vi "TryUpdateAccelerometerSample.vi"   [LabVIEW 2016]
uses:
  <vilib>/Platform/TimedLoop/XDataNode/timing_clust.ctl
  <vilib>/Platform/TimedLoop/XDataNode/nitl_modes.ctl
  <vilib>/Platform/TimedLoop/XDataNode/wakeup.ctl
  Telemetry/TelemetryDataTypes.ctl
  Telemetry/TelemetryUpdateModes.ctl
  Telemetry/TelemetryFields.ctl
  <vilib>/rvi/Emulation/niFpgaEmulationIsFPGAContextNoSignature.vi
  <vilib>/rvi/Emulation/niFpgaSctlEmulationGetInTimedLoop.vi
  <vilib>/rvi/errors/niFpgaSetErrorForExecOnDevCompSimple.vi
  <vilib>/rvi/eio/common/nirviEmuReportErrorAndStop.vi
  <vilib>/rvi/DataTransferAndStorage/Container/Common/niFpgaContainerGetUniqueNameForEmu.vi
  <vilib>/rvi/FIFO/Fifo_Resource/nirvififoEmulationSetSize.vi
  <vilib>/rvi/FIFO/Fifo_Resource/nirviFifoEmulationQueueMgr.vi
  <instcachedir>/0/nirviFifoEmulationQueueMgr_E5CAEC123FF24DC58D834DCA3CDAA9B5.lvgen/nirviFifoEmulationQueueMgr_E5CAEC123FF24DC58D834DCA3CDAA9B5_026.vi
  <vilib>/Utility/error.llb/Clear Errors.vi
  <vilib>/rvi/FIFO/Fifo_Resource/nirvififoEmulationCreateLock.vi
  <vilib>/rvi/Emulation/niFpgaProcessEmulError.vi
  <vilib>/rvi/FIFO/Fifo_Resource/nirvififoEmulationObtainLock.vi
  <vilib>/rvi/FIFO/Fifo_Resource/nirvififoEmulationReleaseLock.vi
  <vilib>/rvi/occurrence/nirviWaitOnOccurrenceBase.vi
  <vilib>/rvi/errors/nirviReportUnexpectedCaseInternalError.vi
  <vilib>/rvi/errors/nirviReportUnexpectedCaseInternalError (U32).vi
  <vilib>/rvi/Emulation/niFpgaEmulationReportErrorSimple.vi
  <vilib>/rvi/Emulation/niFpgaGetClockAttributes.vi
  <vilib>/rvi/Emulation/niFpgaCriticalErrorInLSC.vi
  <instcachedir>/0/nirviFifoEmulationQueueMgr_E5CAEC123FF24DC58D834DCA3CDAA9B5.lvgen/nirviFifoEmulationQueueMgr_E5CAEC123FF24DC58D834DCA3CDAA9B5_038.vi
  <vilib>/rvi/FIFO/Fifo_Resource/nirvififoEmulationDetermineInputValidOut.vi
  <instcachedir>/0/nirviFifoEmulationQueueMgr_E5CAEC123FF24DC58D834DCA3CDAA9B5.lvgen/nirviFifoEmulationQueueMgr_E5CAEC123FF24DC58D834DCA3CDAA9B5_039.vi
  <vilib>/rvi/Memory/Memory_Emulation/niFpgaMemoryEmulationCacheClearOnFirstRun.vi
  <vilib>/rvi/Memory/Memory_Emulation/nirvimemoryEmulationManagerCache_MakeExclusive.vi
  <vilib>/rvi/Memory/Memory_Emulation/niFpgaMemoryEmulationValidateCache.vi
  <vilib>/rvi/Memory/Memory_Emulation/nirvimemoryEmulationManagerCache_InsertValue.vi
  <vilib>/rvi/Memory/Memory_Emulation/nirvimemoryEmulationManagerCache_ReleaseExclusive.vi
  <vilib>/rvi/Memory/Memory_Emulation/nirvimemoryEmulationManagerCache_GetValue.vi
  <vilib>/rvi/Memory/Memory_Emulation/nirvimemoryEmulationManagerCache_SetValue.vi
  <instcachedir>/0/nirviFifoEmulationQueueMgr_E5CAEC123FF24DC58D834DCA3CDAA9B5.lvgen/nirviFifoEmulationQueueMgr_E5CAEC123FF24DC58D834DCA3CDAA9B5_004.vi
  <vilib>/rvi/DataTransferAndStorage/Container/XNode/niFpgaContainer.xnode
  <vilib>/rvi/FIFO/Fifo_Resource/nirvififoEmulationRead.vi
  <vilib>/Platform/TimedLoop/XDataNode/XDataNode.xnode
  <vilib>/rvi/FIFO/Fifo_Resource/nirvififoEmulationWrite.vi
  <vilib>/rvi/DataTransferAndStorage/Register/Emulation/niFpgaRegisterEmulation.vi
  <vilib>/Platform/TimedLoop/XDataNode/XDNodeRunTimeDep.lvlib
types:
  T1 = cluster{"Timestamp":u64, "Accelerometer1Voltage":sgl, "Accelerometer2Voltage":sgl, "Accelerometer3Voltage":sgl, "Accelerometer4Voltage":sgl, "Accelerometer5Voltage":sgl, "Accelerometer6Voltage":sgl, "Accelerometer7Voltage":sgl, "Accelerometer8Voltage":sgl, "Accelerometer1Acceleration":sgl, "Accelerometer2Acceleration":sgl, "Accelerometer3Acceleration":sgl, "Accelerometer4Acceleration":sgl, "Accelerometer5Acceleration":sgl, "Accelerometer6Acceleration":sgl, "Accelerometer7Acceleration":sgl, "Accelerometer8Acceleration":sgl, "AngularAccelerationX":sgl, "AngularAccelerationY":sgl, "AngularAccelerationZ":sgl}
  T2 = typedef "TelemetryFields.ctl" = enum16{"None", "InclinometerTxBytes", "InclinometerRxBytes", "InclinometerTxFrames", "InclinometerRxFrames", "InclinometerErrorTimestamp", "InclinometerErrorCode", "InclinometerSampleTimestamp", "InclinometerRawAngle", "InclinometerZenithAngle", "DisplacementTxBytes", "DisplacementRxBytes", "DisplacementTxFrames", "DisplacementRxFrames", "DisplacementErrorTimestamp", "DisplacementErrorCode", "DisplacementSampleTimestamp", "DisplacementRaw1", "DisplacementRaw2", "DisplacementRaw3", "DisplacementRaw4", "DisplacementRaw5", "DisplacementRaw6", "DisplacementRaw7", "DisplacementRaw8", "DisplacementEng1", "DisplacementEng2", "DisplacementEng3", "DisplacementEng4", "DisplacementEng5", "DisplacementEng6", "DisplacementEng7", "DisplacementEng8", "DisplacementPositionX", "DisplacementPositionY", "DisplacementPositionZ", "DisplacementRotationX", "DisplacementRotationY", "DisplacementRotationZ", "AccelerometerSampleCount", "AccelerometerSampleTimestamp", "AccelerometerRaw1", "AccelerometerRaw2", "AccelerometerRaw3", "AccelerometerRaw4", "AccelerometerRaw5", "AccelerometerRaw6", "AccelerometerRaw7", "AccelerometerRaw8", "AccelerometerEng1", "AccelerometerEng2", "AccelerometerEng3", "AccelerometerEng4", "AccelerometerEng5", "AccelerometerEng6", "AccelerometerEng7", "AccelerometerEng8", "AngularAccelerationX", "AngularAccelerationY", "AngularAccelerationZ", "GyroTxBytes", "GyroRxBytes", "GyroTxFrames", "GyroRxFrames", "GyroErrorTimestamp", "GyroErrorCode", "GyroSampleTimestamp", "AngularVelocityX", "AngularVelocityY", "AngularVelocityZ", "GyroStatus", "GyroSequenceNumber", "GyroTemperature", "GyroBITTimestamp", "GyroBIT0", "GyroBIT1", "GyroBIT2", "GyroBIT3", "GyroBIT4", "GyroBIT5", "GyroBIT6", "GyroBIT7"}
  T3 = typedef "TelemetryUpdateModes.ctl" = enum8{"=", "+", "-", "|"}
  T4 = typedef "TelemetryDataTypes.ctl" = enum8{"U8", "U16", "U32", "U64", "I8", "I16", "I32", "I64", "SGL"}
  T5 = typedef "XDNodeRunTimeDep.lvlib/timing_clust.ctl" = cluster{"Expected End [f-1]":u64, "Actual End [f-1]":u64, "Finished Late? [f-1]":bool, "Expected End [i-1]":u64, "Actual End [i-1]":u64, "Finished Late? [i-1]":bool, "Expected Start [i]":u64, "Actual Start [i]":u64, "Expected Start [f]":u64, "Actual Start [f]":u64, "Source Name":string, "Structure Name":string, "Period":i64, "Deadline":i64, "Offset":i64, "Start":i64, "Priority":i32, "Timeout":i32, "Mode":T6, "Wakeup Reason":T7, "Error":errorcluster, "Source Type":string, "Secondary Source Type":string, "Global End Time":u64, "Global Start Time":u64, "Frame Duration":u64, "Iteration Duration":u64, "Assigned CPU":i32, "I/O Scan Engine Mode":u32}
  T6 = typedef "XDNodeRunTimeDep.lvlib/nitl_modes.ctl" = enum32{"No Change", "Process missed periods, maintain original phase", "Discard missed periods, maintain original phase", "Process missed periods, ignore original phase", "Discard missed periods, ignore original phase"}
  T7 = typedef "XDNodeRunTimeDep.lvlib/wakeup.ctl" = enum32{"Normal", "Aborted", "Asynchronous wakeup", "Timing source error", "Timed loop error", "Timeout"}
  T8 = typedef "TelemetryUpdateData.ctl" = cluster{"DataType":T4, "Mode":T3, "Field":T2, "Data":u64}
  T9 = typedef "TelemetryUpdateDataSGL.ctl" = cluster{"Mode":T3, "Field":T2, "Data":sgl}
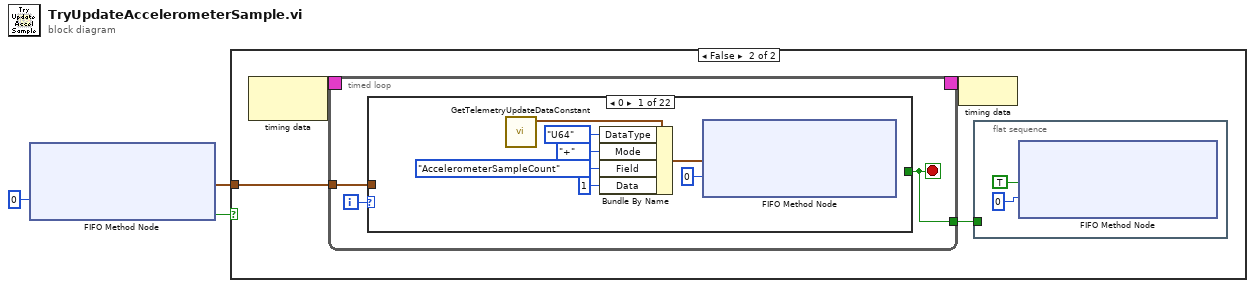
[diagram p0: block diagram]
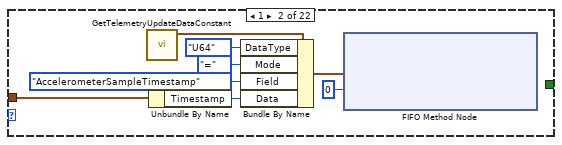
[diagram p3: hidden frame]
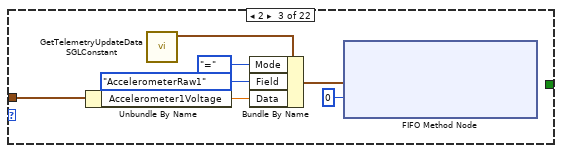
[diagram p4: hidden frame]
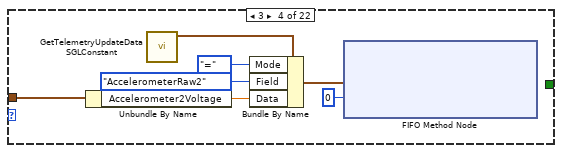
[diagram p5: hidden frame]
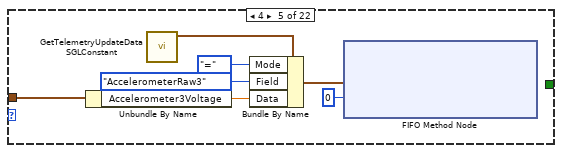
[diagram p6: hidden frame]
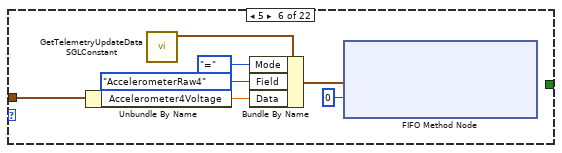
[diagram p7: hidden frame]
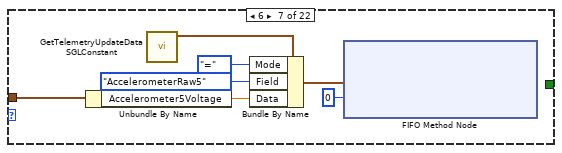
[diagram p8: hidden frame]
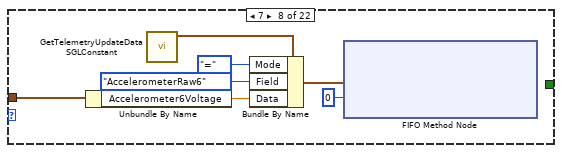
[diagram p9: hidden frame]
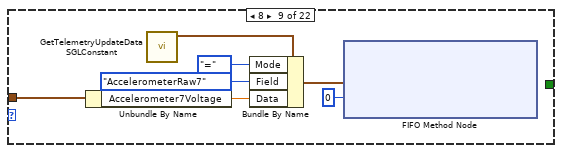
[diagram p10: hidden frame]
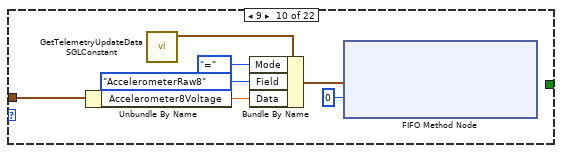
[diagram p11: hidden frame]
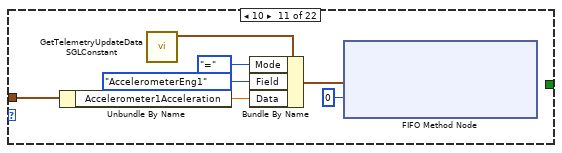
[diagram p12: hidden frame]
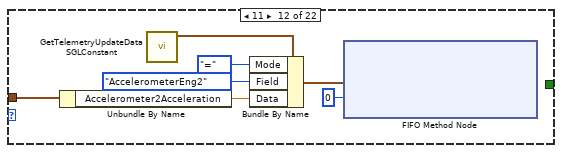
[diagram p13: hidden frame]
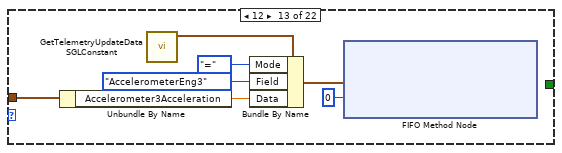
[diagram p14: hidden frame]
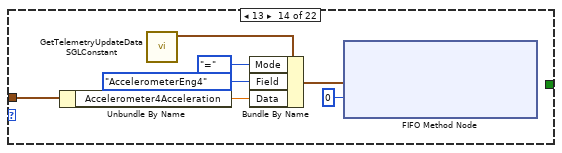
[diagram p15: hidden frame]
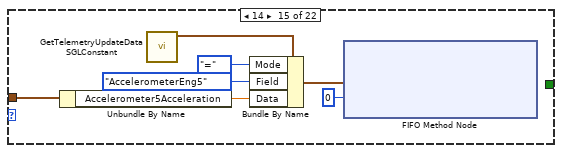
[diagram p16: hidden frame]
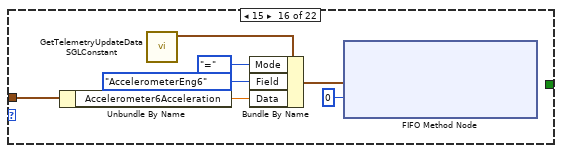
[diagram p17: hidden frame]
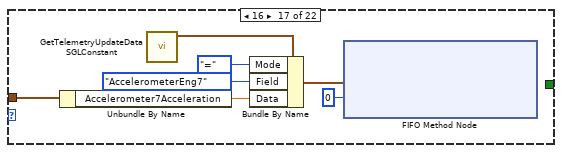
[diagram p18: hidden frame]
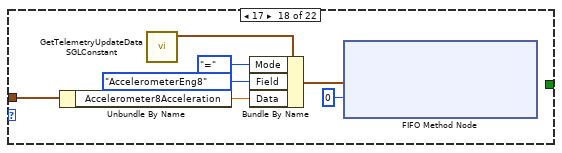
[diagram p19: hidden frame]
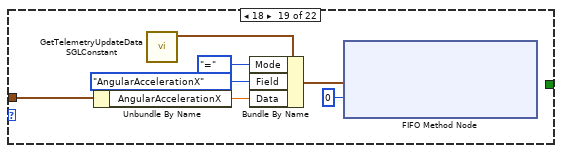
[diagram p20: hidden frame]
diagram:
  n1 = xnode ("FIFO Method Node")("Timeout"=0) -> ("Element"=w2:T1, "Timed Out?"=w3:bool)  [unwired: 1 in, 1 out]
  n2 = case shown="False" w3 {
    tunnel: w2 -> [_ w7]
    frame True {
    }
    frame False {
      n3 = node-c288() -> (w5:T5)  [unwired: 1 in]
      n4 = timed-loop {
        tunnel: w7 -> [w10]
        tunnel: [w9] -> w6
        timing: w5 -> [_]
        timing-out: [_] -> w4
        i -> [w8]
        stop <- w9 stop-if-true
        # "Move Data to Memory"
        n5 = case shown="0" w8 {
          tunnel: w10 -> [_ w19 w27 w34 w41 w48 w55 w62 w69 w76 w83 w90 w97 w104 w111 w118 w125 w132 w139 w146 w153 _]
          tunnel: [_ _ _ _ _ _ _ _ _ _ _ _ _ _ _ _ _ _ _ _ _ w159] -> w9
          frame 0 {
            n6 = call "GetTelemetryUpdateDataConstant.vi"() -> ("TelemetryUpdateData"=w16:T8)  [unwired: 11 in]
            n7 = Bundle By Name(cluster=w16, "DataType"=TelemetryDataTypes."U64" ("TelemetryDataTypes"), "Mode"=TelemetryUpdateModes."+" ("TelemetryUpdateModes"), "Field"=TelemetryFields."AccelerometerSampleCount" ("TelemetryFields"), "Data"=u64 1) -> (w14:T8)
            n8 = xnode ("FIFO Method Node")("Element"=w14, "Timeout"=0) -> ()  [unwired: 1 in, 2 out]
          }
          frame 1 {
            n9 = call "GetTelemetryUpdateDataConstant.vi"() -> ("TelemetryUpdateData"=w25:T8)  [unwired: 11 in]
            n10 = Unbundle By Name(w19) -> ("Timestamp"=w18:u64)
            n11 = Bundle By Name(cluster=w25, "DataType"=TelemetryDataTypes."U64" ("TelemetryDataTypes"), "Mode"=TelemetryUpdateModes."=" ("TelemetryUpdateModes"), "Field"=TelemetryFields."AccelerometerSampleTimestamp" ("TelemetryFields"), "Data"=w18) -> (w23:T8)
            n12 = xnode ("FIFO Method Node")("Element"=w23, "Timeout"=0) -> ()  [unwired: 1 in, 2 out]
          }
          frame 2 {
            n13 = Unbundle By Name(w27) -> ("Accelerometer1Voltage"=w26:sgl)
            n14 = call "GetTelemetryUpdateDataSGLConstant.vi"() -> ("TelemetryUpdateDataSGL"=w32:T9)  [unwired: 11 in]
            n15 = Bundle By Name(cluster=w32, "Mode"=TelemetryUpdateModes."=" ("TelemetryUpdateModes"), "Field"=TelemetryFields."AccelerometerRaw1" ("TelemetryFields"), "Data"=w26) -> (w30:T9)
            n16 = xnode ("FIFO Method Node")("Element"=w30, "Timeout"=0) -> ()  [unwired: 1 in, 2 out]
          }
          frame 3 {
            n17 = Unbundle By Name(w34) -> ("Accelerometer2Voltage"=w33:sgl)
            n18 = call "GetTelemetryUpdateDataSGLConstant.vi"() -> ("TelemetryUpdateDataSGL"=w39:T9)  [unwired: 11 in]
            n19 = Bundle By Name(cluster=w39, "Mode"=TelemetryUpdateModes."=" ("TelemetryUpdateModes"), "Field"=TelemetryFields."AccelerometerRaw2" ("TelemetryFields"), "Data"=w33) -> (w37:T9)
            n20 = xnode ("FIFO Method Node")("Element"=w37, "Timeout"=0) -> ()  [unwired: 1 in, 2 out]
          }
          frame 4 {
            n21 = Unbundle By Name(w41) -> ("Accelerometer3Voltage"=w40:sgl)
            n22 = call "GetTelemetryUpdateDataSGLConstant.vi"() -> ("TelemetryUpdateDataSGL"=w46:T9)  [unwired: 11 in]
            n23 = Bundle By Name(cluster=w46, "Mode"=TelemetryUpdateModes."=" ("TelemetryUpdateModes"), "Field"=TelemetryFields."AccelerometerRaw3" ("TelemetryFields"), "Data"=w40) -> (w44:T9)
            n24 = xnode ("FIFO Method Node")("Element"=w44, "Timeout"=0) -> ()  [unwired: 1 in, 2 out]
          }
          frame 5 {
            n25 = Unbundle By Name(w48) -> ("Accelerometer4Voltage"=w47:sgl)
            n26 = call "GetTelemetryUpdateDataSGLConstant.vi"() -> ("TelemetryUpdateDataSGL"=w53:T9)  [unwired: 11 in]
            n27 = Bundle By Name(cluster=w53, "Mode"=TelemetryUpdateModes."=" ("TelemetryUpdateModes"), "Field"=TelemetryFields."AccelerometerRaw4" ("TelemetryFields"), "Data"=w47) -> (w51:T9)
            n28 = xnode ("FIFO Method Node")("Element"=w51, "Timeout"=0) -> ()  [unwired: 1 in, 2 out]
          }
          frame 6 {
            n29 = Unbundle By Name(w55) -> ("Accelerometer5Voltage"=w54:sgl)
            n30 = call "GetTelemetryUpdateDataSGLConstant.vi"() -> ("TelemetryUpdateDataSGL"=w60:T9)  [unwired: 11 in]
            n31 = Bundle By Name(cluster=w60, "Mode"=TelemetryUpdateModes."=" ("TelemetryUpdateModes"), "Field"=TelemetryFields."AccelerometerRaw5" ("TelemetryFields"), "Data"=w54) -> (w58:T9)
            n32 = xnode ("FIFO Method Node")("Element"=w58, "Timeout"=0) -> ()  [unwired: 1 in, 2 out]
          }
          frame 7 {
            n33 = Unbundle By Name(w62) -> ("Accelerometer6Voltage"=w61:sgl)
            n34 = call "GetTelemetryUpdateDataSGLConstant.vi"() -> ("TelemetryUpdateDataSGL"=w67:T9)  [unwired: 11 in]
            n35 = Bundle By Name(cluster=w67, "Mode"=TelemetryUpdateModes."=" ("TelemetryUpdateModes"), "Field"=TelemetryFields."AccelerometerRaw6" ("TelemetryFields"), "Data"=w61) -> (w65:T9)
            n36 = xnode ("FIFO Method Node")("Element"=w65, "Timeout"=0) -> ()  [unwired: 1 in, 2 out]
          }
          frame 8 {
            n37 = Unbundle By Name(w69) -> ("Accelerometer7Voltage"=w68:sgl)
            n38 = call "GetTelemetryUpdateDataSGLConstant.vi"() -> ("TelemetryUpdateDataSGL"=w74:T9)  [unwired: 11 in]
            n39 = Bundle By Name(cluster=w74, "Mode"=TelemetryUpdateModes."=" ("TelemetryUpdateModes"), "Field"=TelemetryFields."AccelerometerRaw7" ("TelemetryFields"), "Data"=w68) -> (w72:T9)
            n40 = xnode ("FIFO Method Node")("Element"=w72, "Timeout"=0) -> ()  [unwired: 1 in, 2 out]
          }
          frame 9 {
            n41 = Unbundle By Name(w76) -> ("Accelerometer8Voltage"=w75:sgl)
            n42 = call "GetTelemetryUpdateDataSGLConstant.vi"() -> ("TelemetryUpdateDataSGL"=w81:T9)  [unwired: 11 in]
            n43 = Bundle By Name(cluster=w81, "Mode"=TelemetryUpdateModes."=" ("TelemetryUpdateModes"), "Field"=TelemetryFields."AccelerometerRaw8" ("TelemetryFields"), "Data"=w75) -> (w79:T9)
            n44 = xnode ("FIFO Method Node")("Element"=w79, "Timeout"=0) -> ()  [unwired: 1 in, 2 out]
          }
          frame 10 {
            n45 = Unbundle By Name(w83) -> ("Accelerometer1Acceleration"=w82:sgl)
            n46 = call "GetTelemetryUpdateDataSGLConstant.vi"() -> ("TelemetryUpdateDataSGL"=w88:T9)  [unwired: 11 in]
            n47 = Bundle By Name(cluster=w88, "Mode"=TelemetryUpdateModes."=" ("TelemetryUpdateModes"), "Field"=TelemetryFields."AccelerometerEng1" ("TelemetryFields"), "Data"=w82) -> (w86:T9)
            n48 = xnode ("FIFO Method Node")("Element"=w86, "Timeout"=0) -> ()  [unwired: 1 in, 2 out]
          }
          frame 11 {
            n49 = Unbundle By Name(w90) -> ("Accelerometer2Acceleration"=w89:sgl)
            n50 = call "GetTelemetryUpdateDataSGLConstant.vi"() -> ("TelemetryUpdateDataSGL"=w95:T9)  [unwired: 11 in]
            n51 = Bundle By Name(cluster=w95, "Mode"=TelemetryUpdateModes."=" ("TelemetryUpdateModes"), "Field"=TelemetryFields."AccelerometerEng2" ("TelemetryFields"), "Data"=w89) -> (w93:T9)
            n52 = xnode ("FIFO Method Node")("Element"=w93, "Timeout"=0) -> ()  [unwired: 1 in, 2 out]
          }
          frame 12 {
            n53 = Unbundle By Name(w97) -> ("Accelerometer3Acceleration"=w96:sgl)
            n54 = call "GetTelemetryUpdateDataSGLConstant.vi"() -> ("TelemetryUpdateDataSGL"=w102:T9)  [unwired: 11 in]
            n55 = Bundle By Name(cluster=w102, "Mode"=TelemetryUpdateModes."=" ("TelemetryUpdateModes"), "Field"=TelemetryFields."AccelerometerEng3" ("TelemetryFields"), "Data"=w96) -> (w100:T9)
            n56 = xnode ("FIFO Method Node")("Element"=w100, "Timeout"=0) -> ()  [unwired: 1 in, 2 out]
          }
          frame 13 {
            n57 = Unbundle By Name(w104) -> ("Accelerometer4Acceleration"=w103:sgl)
            n58 = call "GetTelemetryUpdateDataSGLConstant.vi"() -> ("TelemetryUpdateDataSGL"=w109:T9)  [unwired: 11 in]
            n59 = Bundle By Name(cluster=w109, "Mode"=TelemetryUpdateModes."=" ("TelemetryUpdateModes"), "Field"=TelemetryFields."AccelerometerEng4" ("TelemetryFields"), "Data"=w103) -> (w107:T9)
            n60 = xnode ("FIFO Method Node")("Element"=w107, "Timeout"=0) -> ()  [unwired: 1 in, 2 out]
          }
          frame 14 {
            n61 = Unbundle By Name(w111) -> ("Accelerometer5Acceleration"=w110:sgl)
            n62 = call "GetTelemetryUpdateDataSGLConstant.vi"() -> ("TelemetryUpdateDataSGL"=w116:T9)  [unwired: 11 in]
            n63 = Bundle By Name(cluster=w116, "Mode"=TelemetryUpdateModes."=" ("TelemetryUpdateModes"), "Field"=TelemetryFields."AccelerometerEng5" ("TelemetryFields"), "Data"=w110) -> (w114:T9)
            n64 = xnode ("FIFO Method Node")("Element"=w114, "Timeout"=0) -> ()  [unwired: 1 in, 2 out]
          }
          frame 15 {
            n65 = Unbundle By Name(w118) -> ("Accelerometer6Acceleration"=w117:sgl)
            n66 = call "GetTelemetryUpdateDataSGLConstant.vi"() -> ("TelemetryUpdateDataSGL"=w123:T9)  [unwired: 11 in]
            n67 = Bundle By Name(cluster=w123, "Mode"=TelemetryUpdateModes."=" ("TelemetryUpdateModes"), "Field"=TelemetryFields."AccelerometerEng6" ("TelemetryFields"), "Data"=w117) -> (w121:T9)
            n68 = xnode ("FIFO Method Node")("Element"=w121, "Timeout"=0) -> ()  [unwired: 1 in, 2 out]
          }
          frame 16 {
            n69 = Unbundle By Name(w125) -> ("Accelerometer7Acceleration"=w124:sgl)
            n70 = call "GetTelemetryUpdateDataSGLConstant.vi"() -> ("TelemetryUpdateDataSGL"=w130:T9)  [unwired: 11 in]
            n71 = Bundle By Name(cluster=w130, "Mode"=TelemetryUpdateModes."=" ("TelemetryUpdateModes"), "Field"=TelemetryFields."AccelerometerEng7" ("TelemetryFields"), "Data"=w124) -> (w128:T9)
            n72 = xnode ("FIFO Method Node")("Element"=w128, "Timeout"=0) -> ()  [unwired: 1 in, 2 out]
          }
          frame 17 {
            n73 = Unbundle By Name(w132) -> ("Accelerometer8Acceleration"=w131:sgl)
            n74 = call "GetTelemetryUpdateDataSGLConstant.vi"() -> ("TelemetryUpdateDataSGL"=w137:T9)  [unwired: 11 in]
            n75 = Bundle By Name(cluster=w137, "Mode"=TelemetryUpdateModes."=" ("TelemetryUpdateModes"), "Field"=TelemetryFields."AccelerometerEng8" ("TelemetryFields"), "Data"=w131) -> (w135:T9)
            n76 = xnode ("FIFO Method Node")("Element"=w135, "Timeout"=0) -> ()  [unwired: 1 in, 2 out]
          }
          frame 18 {
            n77 = Unbundle By Name(w139) -> ("AngularAccelerationX"=w138:sgl)
            n78 = call "GetTelemetryUpdateDataSGLConstant.vi"() -> ("TelemetryUpdateDataSGL"=w144:T9)  [unwired: 11 in]
            n79 = Bundle By Name(cluster=w144, "Mode"=TelemetryUpdateModes."=" ("TelemetryUpdateModes"), "Field"=TelemetryFields."AngularAccelerationX" ("TelemetryFields"), "Data"=w138) -> (w142:T9)
            n80 = xnode ("FIFO Method Node")("Element"=w142, "Timeout"=0) -> ()  [unwired: 1 in, 2 out]
          }
          frame 19 {
            n81 = Unbundle By Name(w146) -> ("AngularAccelerationY"=w145:sgl)
            n82 = call "GetTelemetryUpdateDataSGLConstant.vi"() -> ("TelemetryUpdateDataSGL"=w151:T9)  [unwired: 11 in]
            n83 = Bundle By Name(cluster=w151, "Mode"=TelemetryUpdateModes."=" ("TelemetryUpdateModes"), "Field"=TelemetryFields."AngularAccelerationY" ("TelemetryFields"), "Data"=w145) -> (w149:T9)
            n84 = xnode ("FIFO Method Node")("Element"=w149, "Timeout"=0) -> ()  [unwired: 1 in, 2 out]
          }
          frame 20 {
            n85 = Unbundle By Name(w153) -> ("AngularAccelerationZ"=w152:sgl)
            n86 = call "GetTelemetryUpdateDataSGLConstant.vi"() -> ("TelemetryUpdateDataSGL"=w158:T9)  [unwired: 11 in]
            n87 = Bundle By Name(cluster=w158, "Mode"=TelemetryUpdateModes."=" ("TelemetryUpdateModes"), "Field"=TelemetryFields."AngularAccelerationZ" ("TelemetryFields"), "Data"=w152) -> (w156:T9)
            n88 = xnode ("FIFO Method Node")("Element"=w156, "Timeout"=0) -> ()  [unwired: 1 in, 2 out]
          }
          frame 21, Default {
            n89 = xnode ("Register Read")() -> ("Data"=w159:bool)  [unwired: 1 in, 1 out]
          }
        }
      }
      n90 = node-c288(w4) -> ()
      n91 = flat-sequence {
        tunnel: w6 -> [_]
        frame #0 {
          n92 = xnode ("FIFO Method Node")("Element"=TRUE, "Timeout"=0) -> ()  [unwired: 1 in, 2 out]
        }
      }
    }
  }
